vi "Get ECAT IOVar Data.vi"(8 "Fehler (Eingang, kein Fehler)":errorcluster, 10 "ECAT Variablenobjekt":refnum<k21>[](array[refnum]), 11 "VS ref":T5=18446744073709551615 format="%.0x") -> (0 "Fehler (Ausgang)":errorcluster, 1 "I/O Output Vars":T6[](array[typedef]) {"VS ref" format="%.0x"}, 2 "I/O Imput Vars":T6[](array[typedef]) {"VS ref" format="%.0x"}, 3 "VS ref 2":T5=18446744073709551615 format="%.0x", 5 "I/O Output Data":T1 {"BD Refs"."Data Reference" format="%.0x"}, 7 "I/O Input Data":T4 {"BD Refs"."Data Reference" format="%.0x"})   [LabVIEW 2019, in "SEECD Engine.lvlib"]
uses:
  SEECD Engine.lvlib
  Type Defs/Generic ECAT Slave IOV Cluster.ctl
  <vilib>/NI VeriStand/Custom Device API/Custom Device Item Ref.ctl
  Shared/Type Defs/UDV Data Type.ctl
  Type Defs/Input Data.ctl
  <vilib>/NI VeriStand/Custom Device API/Block Data Reference.ctl
  <vilib>/NI VeriStand/Custom Device API/Data Reference.ctl
  Type Defs/Output Data.ctl
  <vilib>/NI VeriStand/Custom Device API/Data Access Type.ctl
  Type Defs/Data Ref FGV Command.ctl
  Shared/Globals/Property Strings.vi
  Shared/SEECD Shared.lvlib
  <vilib>/NI VeriStand/Custom Device API/Custom Device API.lvlib
  <resource>/objmgr/ni.var.rc
  System Explorer/SEECD System Explorer.lvlib
  <vilib>/NI VeriStand/Custom Device Tools/Custom Device Utility Library/Custom Device Utility Library.lvlib
panel:
  out "ECAT Variablenobjekt out":refnum<k21>[](array[refnum])
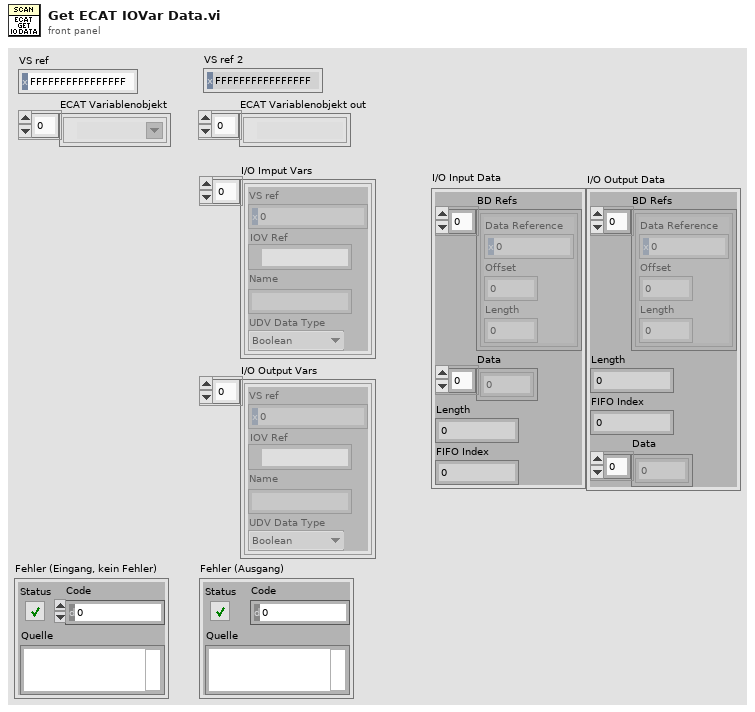
[diagram p1: front panel]
types:
  T1 = typedef "SEECD Engine.lvlib/Output Data.ctl" = cluster{"BD Refs":T2[], "Length":i32, "FIFO Index":i32, "Data":dbl[]}
  T2 = typedef "Custom Device API.lvlib/Block Data Reference.ctl" = cluster{"Data Reference":T3, "Offset":u64, "Length":u64}
  T3 = typedef "Custom Device API.lvlib/Data Reference.ctl" = i32
  T4 = typedef "SEECD Engine.lvlib/Input Data.ctl" = cluster{"BD Refs":T2[], "Data":dbl[], "Length":i32, "FIFO Index":i32}
  T5 = typedef "Custom Device API.lvlib/Custom Device Item Ref.ctl" = u64
  T6 = typedef "SEECD Engine.lvlib/Generic ECAT Slave IOV Cluster.ctl" = cluster{"VS ref":T5, "IOV Ref":refnum<k21>, "Name":string, "UDV Data Type":T7}
  T7 = typedef "SEECD Shared.lvlib/UDV Data Type.ctl" = enum16{"Boolean", "Fixed Point", "Int8", "Int16", "Int32", "Int64", "U32 Bit Field", "UInt8", "UInt16", "UInt32", "UInt64", "Other", "DBL", "SGL"}
  T8 = typedef "SEECD Engine.lvlib/Data Ref FGV Command.ctl" = enum16{"Intialize", "Get", "Update"}
  T9 = typedef "Custom Device API.lvlib/Data Access Type.ctl" = enum16{"Read", "Write"}
  T10 = typedef "SEECD System Explorer.lvlib/ECAT Channel Data Type.ctl" = enum16{"Boolean", "Fixed Point", "Int8", "Int16", "Int32", "Int64", "U32 Bit Field", "UInt8", "UInt16", "UInt32", "UInt64", "Other", "DBL", "SGL"}
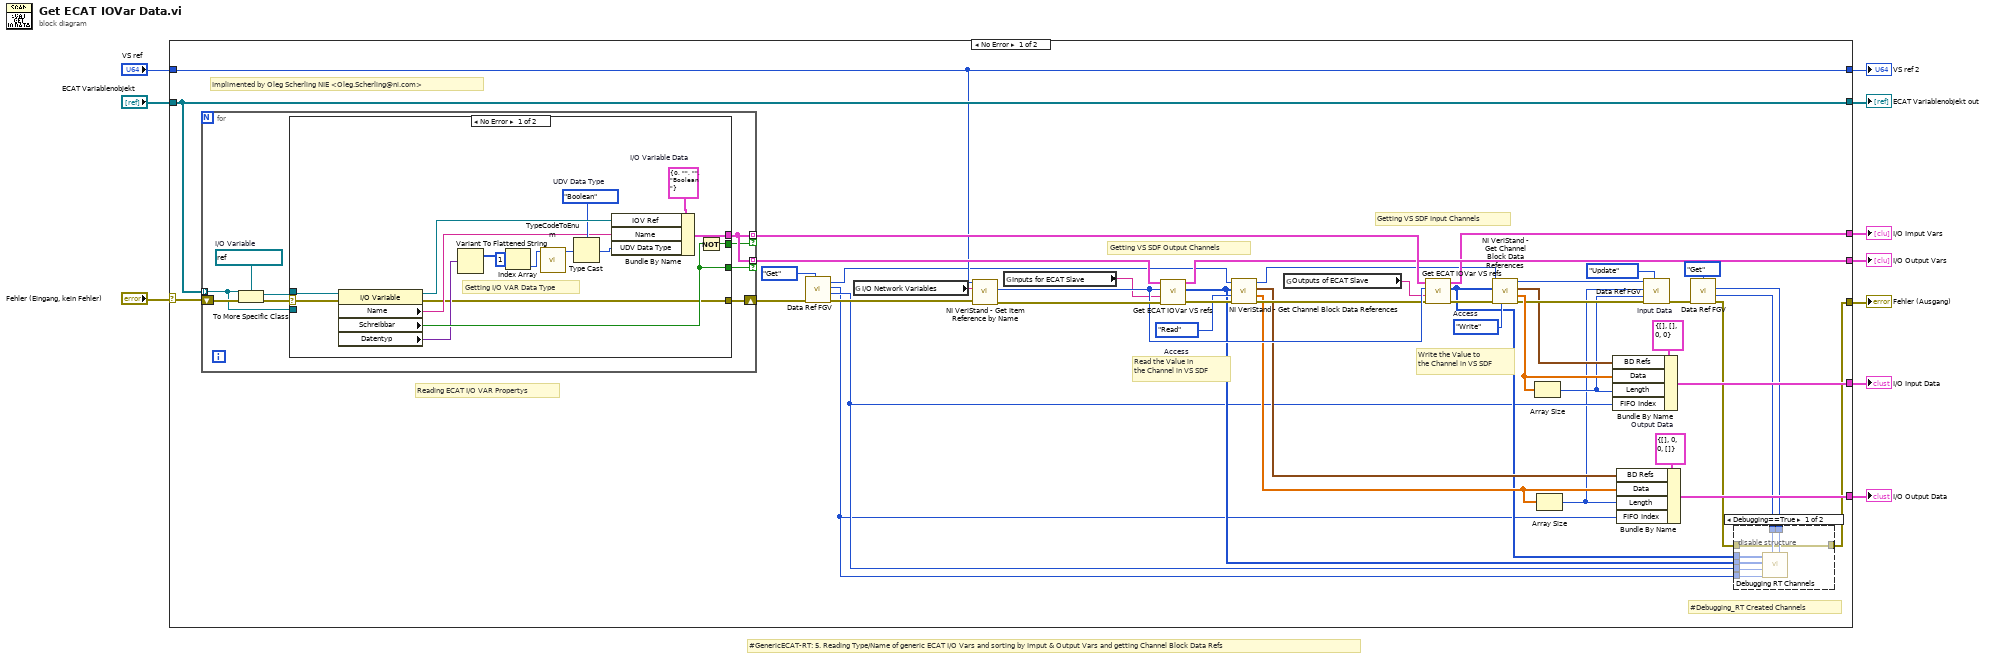
[diagram p0: block diagram]
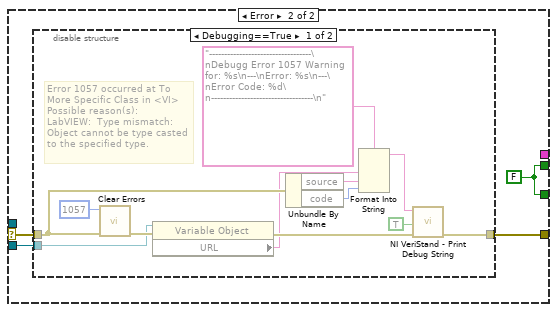
[diagram p2: hidden frame]
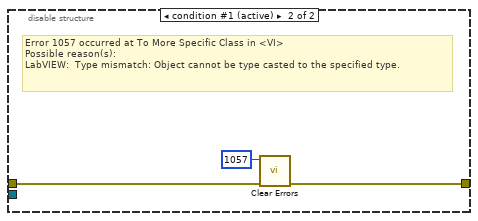
[diagram p3: hidden frame]
diagram:
  # "#GenericECAT-RT: 5. Reading Type/Name of generic ECAT I/O Vars and sorting by Imput & Output Vars and getting Channel Block Data Refs"
  n1 = case shown="No Error" "Fehler (Eingang, kein Fehler)" {
    selector: "Fehler (Eingang, kein Fehler)" -> [w53 w110]
    tunnel: "ECAT Variablenobjekt" -> [w55 w109]
    tunnel: [w15 w110] -> w8
    tunnel: [w55 w109] -> w7
    tunnel: "VS ref" -> [w41 w108]
    tunnel: [w49 _] -> w5
    tunnel: [w48 _] -> w4
    tunnel: [w41 w108] -> w3
    tunnel: [w38 _] -> w2
    tunnel: [w37 _] -> w1
    frame No Error {
      w39 = T1 {"BD Refs"=[], "Length"=0, "FIFO Index"=0, "Data"=[]}  # Output Data
      w40 = T4 {"BD Refs"=[], "Data"=[], "Length"=0, "FIFO Index"=0}  # Input Data
      w43 = Data_Access_Type."Write"  # Access
      w45 = Data_Access_Type."Read"  # Access
      # "Implimented by Oleg Scherling NIE <Oleg.Scherling@ni.com>"
      # "#Debugging_RT Created Channels"
      # "Getting VS SDF Input Channels"
      # "Getting VS SDF Output Channels"
      # "Reading ECAT I/O VAR Propertys"
      # "Write the Value to\nthe Channel in VS SDF"
      # "Read the Value in\nthe Channel in VS SDF"
      n2 = for {
        shift-right: [w59] -> w34
        shift-left: w53 -> [w58]
        tunnel: w55 -> [w56] mode=indexing
        tunnel: [w64] -> w50 mode=indexing if=w63
        tunnel: [w64] -> w54 mode=indexing if=w62
        w61 = refnum<k21> refnum  # I/O Variable
        n3 = To More Specific Class(target class=w61, reference=w56, error in=w58) -> (specific class reference=w60:refnum<k21>, error out=w57:errorcluster)
        n4 = case shown="No Error" w57 {
          selector: w57 -> [w65 w83]
          tunnel: [w78 _] -> w64
          tunnel: [w77 w84] -> w63
          tunnel: [w76 w84] -> w62
          tunnel: w60 -> [w75 _]
          tunnel: [w66 w82] -> w59
          tunnel: w56 -> [_ w81]
          frame No Error {
            w70 = UDV_Data_Type."Boolean"  # UDV Data Type
            w80 = T6 {"VS ref"=0, "IOV Ref"="", "Name"="", "UDV Data Type"=enum."Boolean"}  # I/O Variable Data
            # "Getting I/O VAR Data Type"
            n5 = property class="I/O Variable"(reference=w75, error in=w65) -> (reference out=w79:refnum<k21>, error out=w66:errorcluster, "Name"=w68:string, "Schreibbar"=w76:bool, "Datentyp"=w72:variant)
            n6 = Variant To Flattened String(Variant=w72) -> (1:w73:i16[])  [unwired: 1 out]
            n7 = Index Array(array=w73, index=1) -> (element=w71:i16)
            n8 = call "TypeCodeToEnum.vi"("Type Code (numbers in hexadecimal)"=w71) -> ("UDV Data Type"=w69:T10)  [unwired: 9 in, 1 out]
            n9 = Type Cast(type=w70, x=w69) -> (*(type *) &x=w67:T7)
            n10 = Bundle By Name(cluster=w80, "IOV Ref"=w79, "Name"=w68, "UDV Data Type"=w67) -> (w78:T6)
            n11 = Not(x=w76) -> (.not. x?=w77:bool)
          }
          frame Error {
            w84 = FALSE
            n12 = disable-structure shown="Debugging==True" {
              disable-tunnel: w83 -> [w93 w98]
              disable-tunnel: [w90 w97] -> w82
              disable-tunnel: w81 -> [w89 _]
              frame condition #0 {
                # "Error 1057 occurred at To More Specific Class in <VI>\nPossible reason(s):\nLabVIEW:  Type mismatch: Object cannot be type casted to the specified type."
                n13 = call <vilib>:"Clear Errors.vi"("error in (no error)"=w93, "specific error code to clear (0: all)"=1057) -> ("error out"=w92:errorcluster)  [unwired: 4 in, 1 out]
                n14 = property class="Variable Object"(reference=w89, error in=w92) -> (error out=w91:errorcluster, "URL"=w88:string)  [unwired: 1 out]
                n15 = Unbundle By Name(w93) -> ("source"=w87:string, "code"=w86:i32)
                n16 = Format Into String(format string="----------------------------------\nDebugg Error 1057 Warning for: %s\n---\nError: %s\n---\nError Code: %d\n----------------------------------\n" ("Format-String"), w88, w87, w86) -> (resulting string=w94:string)  [unwired: 2 in, 1 out]
                n17 = call <vilib>:"NI VeriStand - Print Debug String.vi"("error in (no error)"=w91, "Add to log file? (F)"=TRUE, "Message"=w94) -> ("error out"=w90:errorcluster)  [unwired: 8 in]
              }
              frame condition #1 (active) {
                # "Error 1057 occurred at To More Specific Class in <VI>\nPossible reason(s):\nLabVIEW:  Type mismatch: Object cannot be type casted to the specified type."
                n18 = call <vilib>:"Clear Errors.vi"("error in (no error)"=w98, "specific error code to clear (0: all)"=1057) -> ("error out"=w97:errorcluster)  [unwired: 4 in, 1 out]
              }
            }
          }
        }
      }
      n19 = call "Data Ref FGV.vi"("Command"=Data_Ref_FGV_Command."Get", "error in (no error)"=w34) -> ("error out"=w33:errorcluster, "Output FIFO Index / Length"=w14:i32, "Input FIFO Index / Length"=w13:i32, "Device Ref out"=w23:T5)  [unwired: 6 in]
      n20 = global read "Property Strings.vi" "I/O Network Variables"() -> (w52:string)
      n21 = call <vilib>:"NI VeriStand - Get Item Reference by Name.vi"("error in (no error)"=w33, "Item Name"=w52, "Parent Ref in"=w41) -> ("error out"=w51:errorcluster, "Item Ref"=w47:T5)  [unwired: 5 in, 2 out]
      n22 = global read "Property Strings.vi" "Inputs for ECAT Slave"() -> (w29:string)
      n23 = call "Get ECAT IOVar VS refs.vi"("Fehler (Eingang, kein Fehler)"=w51, "Section Name"=w29, "Item Ref"=w47, "I/O Variable Data in"=w54) -> ("Fehler (Ausgang)"=w46:errorcluster, "Channel Refs"=w19:T5[], "I/O Variable Data out"=w49:T6[])  [unwired: 5 in]
      n24 = call <vilib>:"NI VeriStand - Get Channel Block Data References.vi"("error in (no error)"=w46, "Access"=w45, "Channel Refs"=w19, "Device Ref in"=w23) -> ("error out"=w44:errorcluster, "Values Array"=w27:dbl[], "Block Data Refs"=w25:T2[], "Device Ref out"=w24:T5)  [unwired: 4 in]
      n25 = global read "Property Strings.vi" "Outputs of ECAT Slave"() -> (w28:string)
      n26 = call "Get ECAT IOVar VS refs.vi"("Fehler (Eingang, kein Fehler)"=w44, "Section Name"=w28, "Item Ref"=w47, "I/O Variable Data in"=w50) -> ("Fehler (Ausgang)"=w42:errorcluster, "Channel Refs"=w20:T5[], "I/O Variable Data out"=w48:T6[])  [unwired: 5 in]
      n27 = call <vilib>:"NI VeriStand - Get Channel Block Data References.vi"("error in (no error)"=w42, "Access"=w43, "Channel Refs"=w20, "Device Ref in"=w24) -> ("error out"=w32:errorcluster, "Values Array"=w35:dbl[], "Block Data Refs"=w26:T2[], "Device Ref out"=w30:T5)  [unwired: 4 in]
      n28 = Array Size(array=w35) -> (size(s)=w12:i32)
      n29 = Array Size(array=w27) -> (size(s)=w11:i32)
      n30 = Bundle By Name(cluster=w40, "BD Refs"=w26, "Data"=w35, "Length"=w12, "FIFO Index"=w14) -> (w38:T4)
      n31 = Bundle By Name(cluster=w39, "BD Refs"=w25, "Data"=w27, "Length"=w11, "FIFO Index"=w13) -> (w37:T1)
      n32 = call "Data Ref FGV.vi"("Command"=Data_Ref_FGV_Command."Update", "error in (no error)"=w32, "Output Length"=w12, "Input Length"=w11, "Device Ref in"=w30) -> ("error out"=w22:errorcluster)  [unwired: 3 in, 3 out]
      n33 = call "Data Ref FGV.vi"("Command"=Data_Ref_FGV_Command."Get", "error in (no error)"=w22) -> ("error out"=w16:errorcluster, "Output FIFO Index / Length"=w18:i32, "Input FIFO Index / Length"=w17:i32)  [unwired: 6 in, 1 out]
      n34 = disable-structure shown="Debugging==True" {
        disable-tunnel: w20 -> [w106 _]
        disable-tunnel: w19 -> [w105 _]
        disable-tunnel: w18 -> [w104 _]
        disable-tunnel: w17 -> [w103 _]
        disable-tunnel: w16 -> [w102 w107]
        disable-tunnel: [w102 w107] -> w15
        disable-tunnel: w13 -> [w101 _]
        disable-tunnel: w14 -> [w100 _]
        frame condition #0 {
          n35 = call "Debugging RT Channels.vi"("Output FIFO Length"=w103, "Input FIFO Length"=w104, "Output FIFO Index"=w101, "Input FIFO Index"=w100, "Output  Channel Refs"=w105, "Input Channel Refs"=w106) -> ()  [unwired: 6 in]
        }
        frame condition #1 (active) {
        }
      }
    }
    frame Error {
    }
  }
  "I/O Imput Vars" <- w4
  "I/O Output Vars" <- w5
  "Fehler (Ausgang)" <- w8
  "ECAT Variablenobjekt out" <- w7
  "VS ref 2" <- w3
  "I/O Input Data" <- w2
  "I/O Output Data" <- w1
